vi "dynEinheiten.vi"(8 "Komponenten Ref.":refnum<vi>[](array[refnum]), 9 "max.Abweichung Ref.":refnum<vi>[](array[refnum]), 10 "Sollwert Ref.":refnum<vi>[](array[refnum]), 11 "Istwerte Ref.":refnum<vi>[](array[refnum])) -> ()   [LabVIEW 2020, in "EPA 1065.lvlib" / "Interference verificaton 1065-366.lvlib"]
uses:
  Interference verificaton 1065-366.lvlib
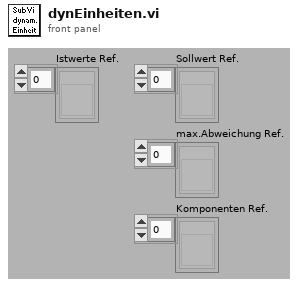
[diagram p1: front panel]
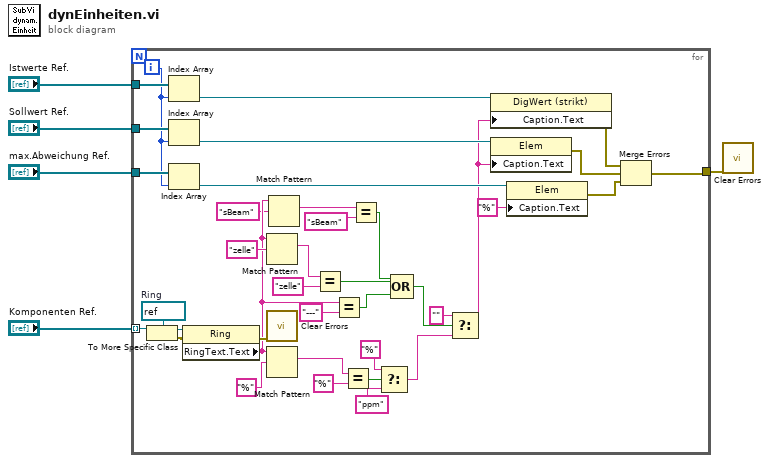
[diagram p0: block diagram]
diagram:
  n1 = for {
    tunnel: "Sollwert Ref." -> [w42]
    tunnel: "max.Abweichung Ref." -> [w41]
    tunnel: "Istwerte Ref." -> [w43]
    tunnel: [w33] -> w2
    tunnel: "Komponenten Ref." -> [w7] mode=indexing
    i -> [w40]
    w30 = refnum<vi> refnum  # Ring
    n2 = To More Specific Class(target class=w30, reference=w7) -> (specific class reference=w31:refnum<vi>, error out=w20:errorcluster)  [unwired: 1 in]
    n3 = Index Array(array=w43, index=w40) -> (element=w39:refnum<vi>)
    n4 = Index Array(array=w42, index=w40) -> (element=w38:refnum<vi>)
    n5 = Index Array(array=w41, index=w40) -> (element=w37:refnum<vi>)
    n6 = property class="Ring"(reference=w31, error in=w20) -> (error out=w24:errorcluster, "RingText.Text"=w15:string)  [unwired: 1 out]
    n7 = Match Pattern(string=w15, regular expression="zelle" ("Regulärer Ausdruck")) -> (match substring=w16:string)  [unwired: 1 in, 3 out]
    n8 = call <vilib>:"Clear Errors.vi"("error in (no error)"=w24) -> ()  [unwired: 5 in, 2 out]
    n9 = Match Pattern(string=w15, regular expression="%" ("Nach String/Zeichen suchen (-)")) -> (match substring=w19:string)  [unwired: 1 in, 3 out]
    n10 = Match Pattern(string=w15, regular expression="sBeam" ("Regulärer Ausdruck")) -> (match substring=w12:string)  [unwired: 1 in, 3 out]
    n11 = Equal?(x=w16, y="zelle") -> (x = y?=w10:bool)
    n12 = Equal?(x=w15, y="---") -> (x = y?=w9:bool)
    n13 = Equal?(x=w19, y="%") -> (x = y?=w27:bool)
    n14 = Equal?(x=w12, y="sBeam") -> (x = y?=w11:bool)
    n15 = Select(t="%" ("y"), s=w27, f="ppm") -> (s? t:f=w22:string)
    n16 = Compound Arithmetic op=OR(w11, w10, w9) -> (w8:bool)
    n17 = Select(t="", s=w8, f=w22) -> (s? t:f=w32:string)
    n18 = property class="DigWert (strikt)"(reference=w39, "Caption.Text"=w32) -> (error out=w36:errorcluster)  [unwired: 1 in, 1 out]
    n19 = property class="Elem"(reference=w38, "Caption.Text"=w32) -> (error out=w35:errorcluster)  [unwired: 1 in, 1 out]
    n20 = property class="Elem"(reference=w37, "Caption.Text"="%" ("Untertitel.Text")) -> (error out=w34:errorcluster)  [unwired: 1 in, 1 out]
    n21 = Merge Errors(w36, w35, w34) -> (w33:errorcluster)
  }
  n22 = call <vilib>:"Clear Errors.vi"("error in (no error)"=w2) -> ()  [unwired: 5 in, 2 out]
